vi "IntakeForTime.vi"() -> ()   [LabVIEW 2020]
uses:
  Framework/Robot Global Data.vi
panel:
  in  "NoWait":bool
  in  "Duration":dbl
  in  "WheelsSetpoint":dbl
  in  "TubingSetpoint":dbl
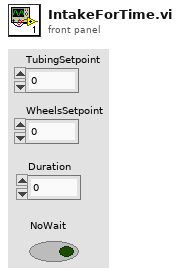
[diagram p1: front panel]
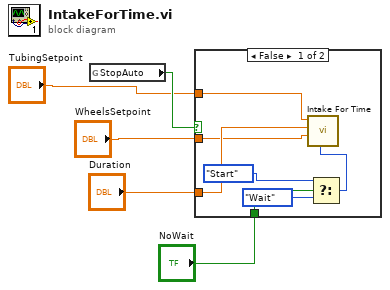
[diagram p0: block diagram]
diagram:
  n1 = global read "Robot Global Data.vi" "StopAuto"() -> (w5:bool)
  n2 = case shown="False" w5 {
    tunnel: "Duration" -> [w12 _]
    tunnel: "WheelsSetpoint" -> [w11 _]
    tunnel: "TubingSetpoint" -> [w10 _]
    tunnel: "NoWait" -> [w9 _]
    frame False {
      n3 = Select(t=enum16{"Start", "Wait"}."Start" ("Synchronization"), s=w9, f=enum16{"Start", "Wait"}."Wait" ("Synchronization")) -> (s? t:f=w6:enum16{"Start", "Wait"})
      n4 = call "Intake For Time.vi"("Synchronization"=w6, "Wheels"=w11, "Duration (s)"=w12, "Tubing"=w10) -> ()  [unwired: 7 in, 1 out]
    }
    frame True {
    }
  }
